vi "Annotations_To_XYgraph.vi"(10 "error in (no error)":errorcluster, 11 "XYGraph in":refnum<vi>) -> (2 "error out":errorcluster, 3 "reference out":refnum<vi>)   [LabVIEW 2017]
uses:
  <vilib>/Utility/miscctls.llb/LVAnnotationListTypeDef.ctl
panel:
  out "Annotation List":T1
  out "AnntList":T1
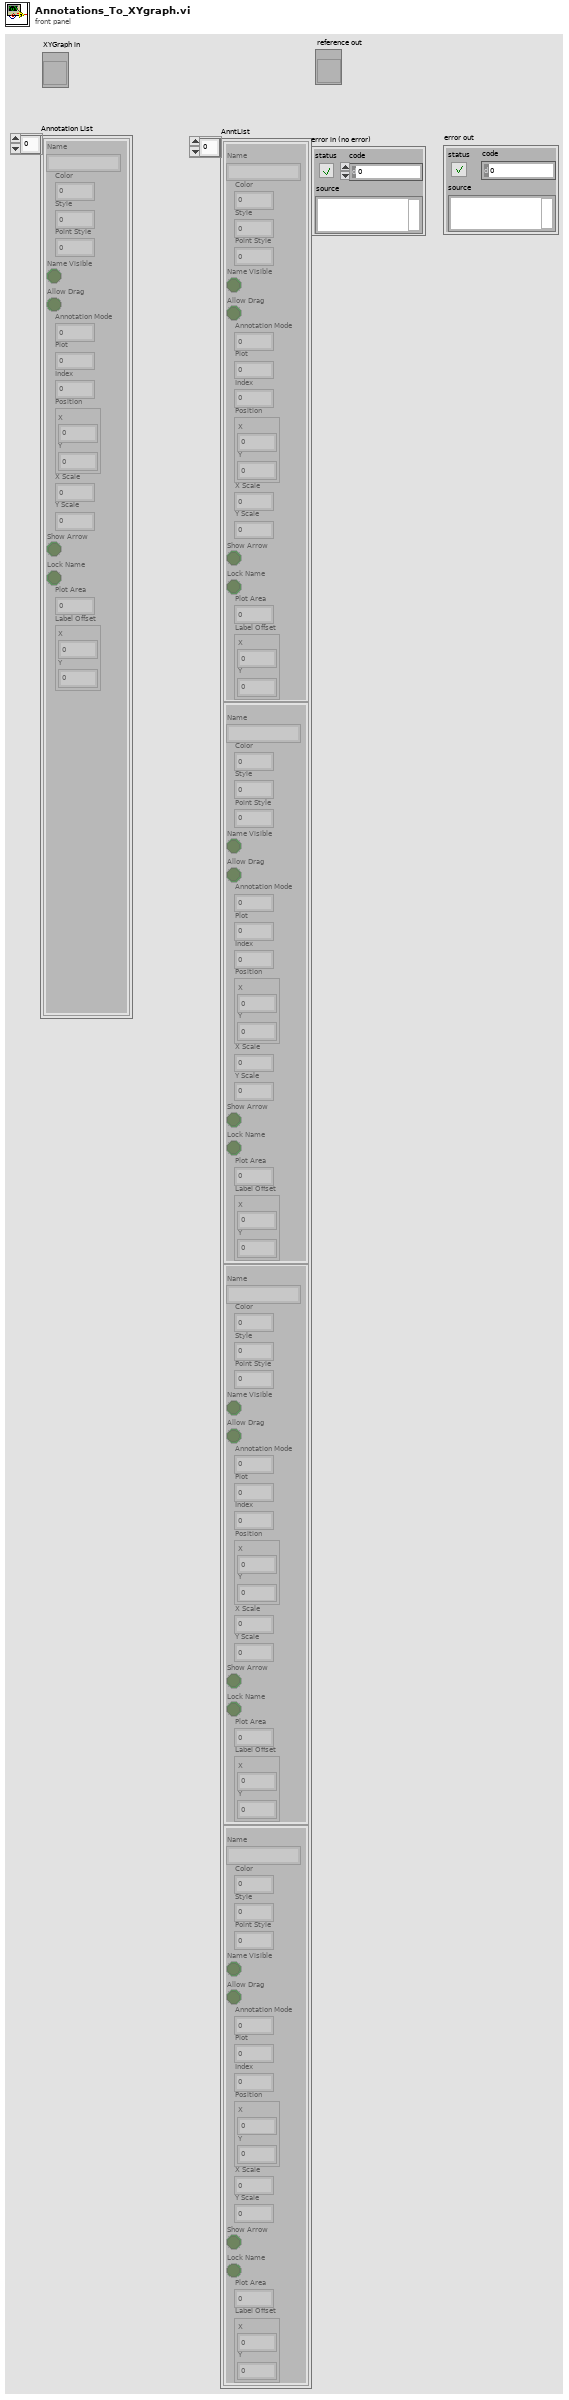
[diagram p1: front panel]
types:
  T1 = typedef "LVAnnotationListTypeDef.ctl" = cluster{"Name":string, "Color":u32, "Style":u8, "Point Style":u8, "Name Visible":bool, "Allow Drag":bool, "Annotation Mode":u32, "Plot":i32, "Index":i32, "Position":cluster{"X":dbl, "Y":dbl}, "X Scale":u32, "Y Scale":u32, "Show Arrow":bool, "Lock Name":bool, "Plot Area":i32, "Label Offset":cluster{"X":dbl, "Y":dbl}}[]
  T2 = cluster{"Name":string, "Color":u32, "Style":u8, "Point Style":u8, "Name Visible":bool, "Allow Drag":bool, "Annotation Mode":u32, "Plot":i32, "Index":i32, "Position":cluster{"X":dbl, "Y":dbl}, "X Scale":u32, "Y Scale":u32, "Show Arrow":bool, "Lock Name":bool, "Plot Area":i32, "Label Offset":cluster{"X":dbl, "Y":dbl}}
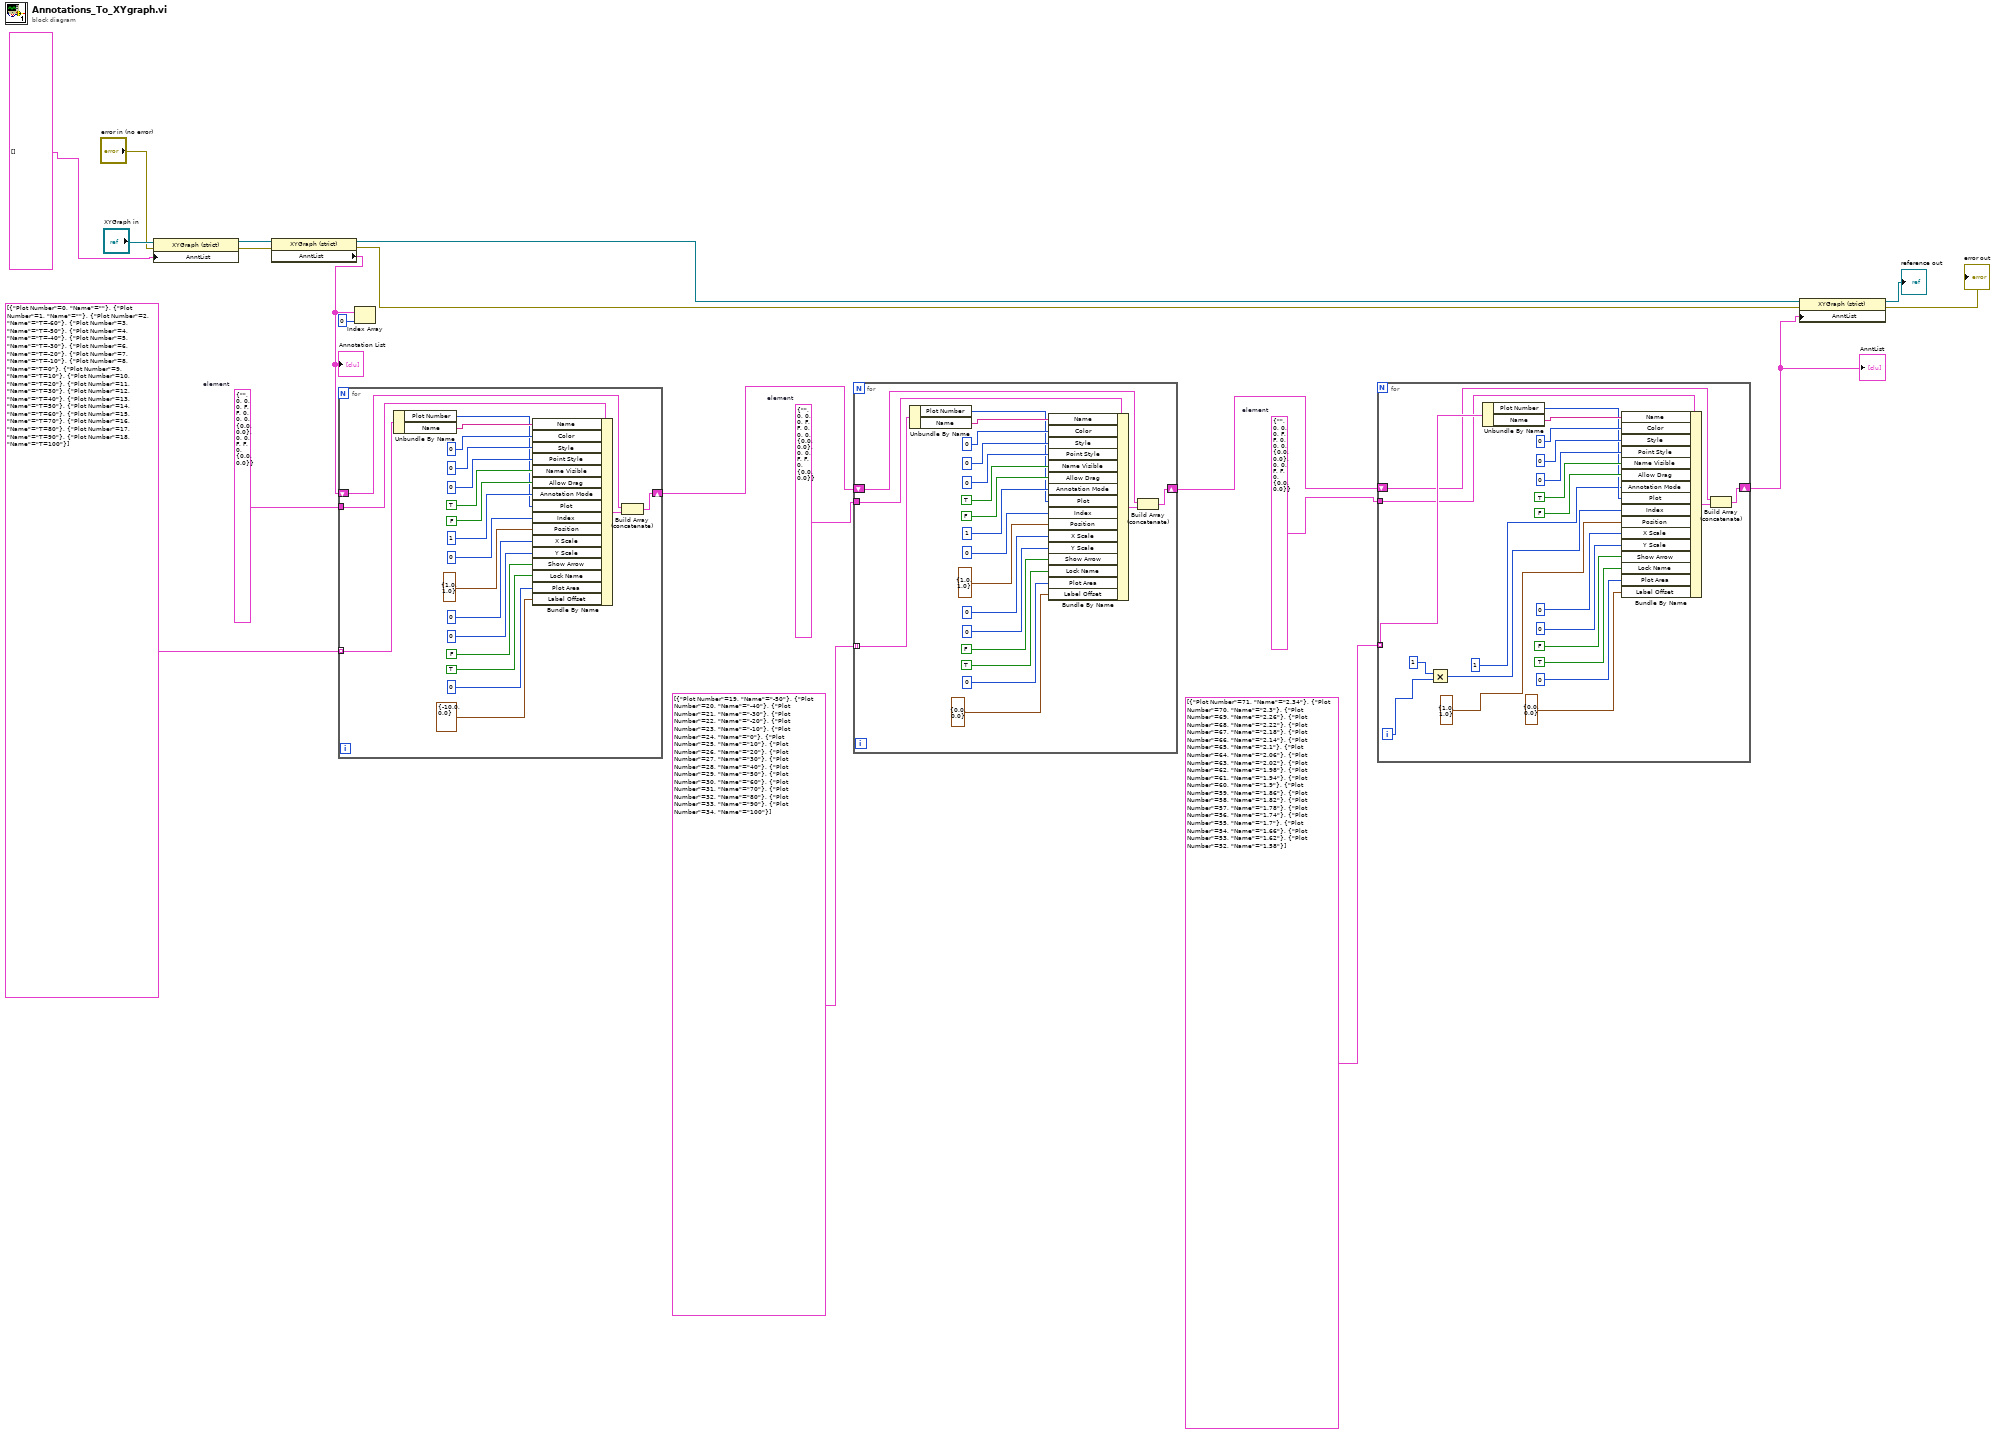
[diagram p0: block diagram]
diagram:
  w3 = T2 {"Name"="", "Color"=0, "Style"=0, "Point Style"=0, "Name Visible"=FALSE, "Allow Drag"=FALSE, "Annotation Mode"=0, "Plot"=0, "Index"=0, "Position"={"X"=0.0, "Y"=0.0}, "X Scale"=0, "Y Scale"=0, "Show Arrow"=FALSE, "Lock Name"=FALSE, "Plot Area"=0, "Label Offset"={"X"=0.0, "Y"=0.0}}  # element
  w15 = T2 {"Name"="", "Color"=0, "Style"=0, "Point Style"=0, "Name Visible"=FALSE, "Allow Drag"=FALSE, "Annotation Mode"=0, "Plot"=0, "Index"=0, "Position"={"X"=0.0, "Y"=0.0}, "X Scale"=0, "Y Scale"=0, "Show Arrow"=FALSE, "Lock Name"=FALSE, "Plot Area"=0, "Label Offset"={"X"=0.0, "Y"=0.0}}  # element
  w20 = T2 {"Name"="", "Color"=0, "Style"=0, "Point Style"=0, "Name Visible"=FALSE, "Allow Drag"=FALSE, "Annotation Mode"=0, "Plot"=0, "Index"=0, "Position"={"X"=0.0, "Y"=0.0}, "X Scale"=0, "Y Scale"=0, "Show Arrow"=FALSE, "Lock Name"=FALSE, "Plot Area"=0, "Label Offset"={"X"=0.0, "Y"=0.0}}  # element
  # "19"
  # "18"
  # "17"
  # "16"
  # "15"
  # "14"
  # "13"
  # "12"
  # "11"
  # "10"
  # "9"
  # "8"
  # "7"
  # "6"
  # "5"
  # "4"
  # "3"
  # "2"
  # "1"
  # "0"
  n1 = property on="Property Node" class="XYGraph (strict)"(reference="XYGraph in", error in="error in (no error)", "AnntList"=T1 [] ("Annotation List")) -> (reference out=w12:refnum<vi>, error out=w7:errorcluster)
  n2 = property on="Property Node" class="XYGraph (strict)"(reference=w12, error in=w7) -> (reference out=w10:refnum<vi>, error out=w6:errorcluster, "AnntList"=w11:T1)
  "Annotation List" <- w11
  n3 = for {
    tunnel: cluster{"Plot Number":i32, "Name":string}[] [{"Plot Number"=0, "Name"=""}, {"Plot Number"=1, "Name"=""}, {"Plot Number"=2, "Name"="T=-60"}, {"Plot Number"=3, "Name"="T=-50"}, {"Plot Number"=4, "Name"="T=-40"}, {"Plot Number"=5, "Name"="T=-30"}, {"Plot Number"=6, "Name"="T=-20"}, {"Plot Number"=7, "Name"="T=-10"}, {"Plot Number"=8, "Name"="T=0"}, {"Plot Number"=9, "Name"="T=10"}, {"Plot Number"=10, "Name"="T=20"}, {"Plot Number"=11, "Name"="T=30"}, {"Plot Number"=12, "Name"="T=40"}, {"Plot Number"=13, "Name"="T=50"}, {"Plot Number"=14, "Name"="T=60"}, {"Plot Number"=15, "Name"="T=70"}, {"Plot Number"=16, "Name"="T=80"}, {"Plot Number"=17, "Name"="T=90"}, {"Plot Number"=18, "Name"="T=100"}] -> [w27] mode=indexing
    tunnel: w20 -> [w24]
    shift-right: [w22] -> w16
    shift-left: w11 -> [w21]
    n4 = Unbundle By Name(w27) -> ("Plot Number"=w25:i32, "Name"=w26:string)
    n5 = Bundle By Name(cluster=w24, "Name"=w26, "Color"=u32 0, "Style"=u8 0, "Point Style"=u8 0, "Name Visible"=TRUE, "Allow Drag"=FALSE, "Annotation Mode"=u32 1, "Plot"=w25, "Index"=0, "Position"=cluster{"X":dbl, "Y":dbl} {"X"=1.0, "Y"=1.0}, "X Scale"=u32 0, "Y Scale"=u32 0, "Show Arrow"=FALSE, "Lock Name"=TRUE, "Plot Area"=0, "Label Offset"=cluster{"X":dbl, "Y":dbl} {"X"=-10.0, "Y"=0.0}) -> (w23:T2)
    n6 = Build Array (concatenate)(w21, w23) -> (w22:T1)
  }
  n7 = Index Array(array=w11, index=0) -> ()  [unwired: 1 out]
  n8 = for {
    tunnel: cluster{"Plot Number":i32, "Name":string}[] [{"Plot Number"=19, "Name"="-50"}, {"Plot Number"=20, "Name"="-40"}, {"Plot Number"=21, "Name"="-30"}, {"Plot Number"=22, "Name"="-20"}, {"Plot Number"=23, "Name"="-10"}, {"Plot Number"=24, "Name"="0"}, {"Plot Number"=25, "Name"="10"}, {"Plot Number"=26, "Name"="20"}, {"Plot Number"=27, "Name"="30"}, {"Plot Number"=28, "Name"="40"}, {"Plot Number"=29, "Name"="50"}, {"Plot Number"=30, "Name"="60"}, {"Plot Number"=31, "Name"="70"}, {"Plot Number"=32, "Name"="80"}, {"Plot Number"=33, "Name"="90"}, {"Plot Number"=34, "Name"="100"}] -> [w48] mode=indexing
    tunnel: w15 -> [w45]
    shift-right: [w43] -> w4
    shift-left: w16 -> [w42]
    n9 = Unbundle By Name(w48) -> ("Plot Number"=w46:i32, "Name"=w47:string)
    n10 = Bundle By Name(cluster=w45, "Name"=w47, "Color"=u32 0, "Style"=u8 0, "Point Style"=u8 0, "Name Visible"=TRUE, "Allow Drag"=FALSE, "Annotation Mode"=u32 1, "Plot"=w46, "Index"=0, "Position"=cluster{"X":dbl, "Y":dbl} {"X"=1.0, "Y"=1.0}, "X Scale"=u32 0, "Y Scale"=u32 0, "Show Arrow"=FALSE, "Lock Name"=TRUE, "Plot Area"=0, "Label Offset"=cluster{"X":dbl, "Y":dbl} {"X"=0.0, "Y"=0.0}) -> (w44:T2)
    n11 = Build Array (concatenate)(w42, w44) -> (w43:T1)
  }
  n12 = for {
    tunnel: cluster{"Plot Number":i32, "Name":string}[] [{"Plot Number"=71, "Name"="2.34"}, {"Plot Number"=70, "Name"="2.3"}, {"Plot Number"=69, "Name"="2.26"}, {"Plot Number"=68, "Name"="2.22"}, {"Plot Number"=67, "Name"="2.18"}, {"Plot Number"=66, "Name"="2.14"}, {"Plot Number"=65, "Name"="2.1"}, {"Plot Number"=64, "Name"="2.06"}, {"Plot Number"=63, "Name"="2.02"}, {"Plot Number"=62, "Name"="1.98"}, {"Plot Number"=61, "Name"="1.94"}, {"Plot Number"=60, "Name"="1.9"}, {"Plot Number"=59, "Name"="1.86"}, {"Plot Number"=58, "Name"="1.82"}, {"Plot Number"=57, "Name"="1.78"}, {"Plot Number"=56, "Name"="1.74"}, {"Plot Number"=55, "Name"="1.7"}, {"Plot Number"=54, "Name"="1.66"}, {"Plot Number"=53, "Name"="1.62"}, {"Plot Number"=52, "Name"="1.58"}] -> [w74] mode=indexing
    tunnel: w3 -> [w71]
    shift-right: [w69] -> w1
    shift-left: w4 -> [w68]
    i -> [w65]
    n13 = Multiply(x=1, y=w65) -> (x*y=w67:i32)
    n14 = Unbundle By Name(w74) -> ("Plot Number"=w72:i32, "Name"=w73:string)
    n15 = Bundle By Name(cluster=w71, "Name"=w73, "Color"=u32 0, "Style"=u8 0, "Point Style"=u8 0, "Name Visible"=TRUE, "Allow Drag"=FALSE, "Annotation Mode"=u32 1, "Plot"=w72, "Index"=w67, "Position"=cluster{"X":dbl, "Y":dbl} {"X"=1.0, "Y"=1.0}, "X Scale"=u32 0, "Y Scale"=u32 0, "Show Arrow"=FALSE, "Lock Name"=TRUE, "Plot Area"=0, "Label Offset"=cluster{"X":dbl, "Y":dbl} {"X"=0.0, "Y"=0.0}) -> (w70:T2)
    n16 = Build Array (concatenate)(w68, w70) -> (w69:T1)
  }
  "AnntList" <- w1
  n17 = property on="Property Node" class="XYGraph (strict)"(reference=w10, error in=w6, "AnntList"=w1) -> (reference out=→"reference out":refnum<vi>, error out=→"error out":errorcluster)
